vi "UniversalCallback.vi"(4 "Request Button":refnum<vi>, 6 "Control Ref":refnum<k24>, 7 "Event Common Data":T1) -> ()   [LabVIEW 2018]
uses:
  Spels.AutomationTools.RemoteFunctionalControlService.dll
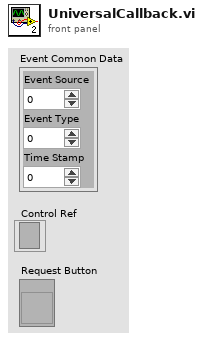
[diagram p1: front panel]
types:
  T1 = cluster{"Event Source":i32, "Event Type":u32, "Time Stamp":u32}
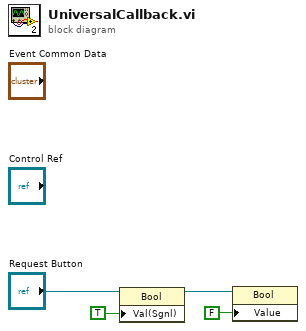
[diagram p0: block diagram]
diagram:
  n1 = property class="Bool"(reference="Request Button", "Val(Sgnl)"=TRUE) -> (reference out=w1:refnum<vi>)  [unwired: 1 in, 1 out]
  n2 = property class="Bool"(reference=w1, "Value"=FALSE) -> ()  [unwired: 1 in, 2 out]
